vi "Send Launch Nested Panel.vi"(4 "Auto-stop? (T)":bool=TRUE, 6 "timeout in ms (-1)":i32=-1, 7 "Priority":T1=enum."Normal" caption="Message Priority (Normal)", 8 "Error In":errorcluster, 9 "Panel":refnum<class "Panel.lvclass">, 10 "Nested Panel Actor":refnum<class "Panel Actor.lvclass">, 11 "Self Enqueuer in":refnum<class "Message Enqueuer.lvclass">) -> (0 "Error Out":errorcluster, 1 "timed out?":bool, 2 "Nested Actor's Enqueuer":refnum<class "Message Enqueuer.lvclass">)   [LabVIEW 2017, in "MGI-Panel Actor.lvlib" / "Panel Actor.lvclass"]
doc: "Sends a message to the actor to launch a nested panel.\n\n<B>Self Enqueuer In:</B> Enqueuer to send the nested panel message\n<B>Nested Panel Actor:</B> Panel actor to launch as a nested actor.\n<B>Panel:</B> Panel object for displaying the nested Panel Actor.\n<B>timeout in ms (-1):</B> Sets the timeout for launching the nested actor\n<B>Message Priority:</B> Sets the priority for the message.\n<B>Auto-Stop?:</B> Defines if the actor should stop automatically.\n<B>Error In:</B> Describes error conditions that occur before this node runs.\n\n<B>Nested Actor's Enqueuer:</B> Enqueuer for the newly spawned nested actor.\n<B>timed out?</B> Indicates if the action timed out.\n<B>Error Out:</B> Contains error information.\n----\nCopyright: MGI 2018\nAuthor: Derek Trepanier"
uses:
  Panel Actor.lvclass
  <vilib>/ActorFramework/Message Enqueuer/Message Enqueuer.lvclass
  <vilib>/ActorFramework/Message Enqueuer/Message Priority.ctl
  panel-manager/Source/Panel/Panel.lvclass
  Panel Actor Messages/Launch Nested Panel Message Msg/Launch Nested Panel Message Msg.lvclass
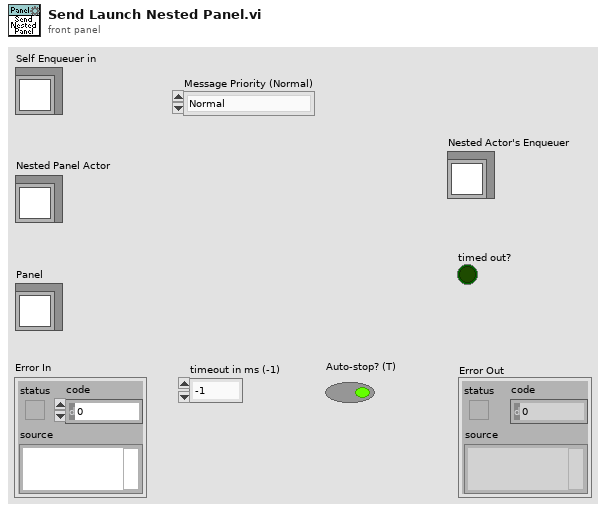
[diagram p1: front panel]
types:
  T1 = typedef "Actor Framework.lvlib/Message Enqueuer.lvclass/Message Priority.ctl" = enum16{"Low", "Normal", "High"}
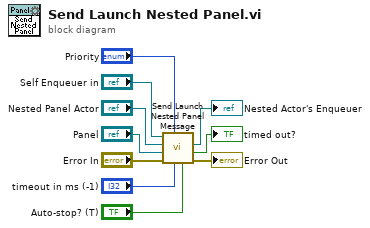
[diagram p0: block diagram]
diagram:
  n1 = call "Send Launch Nested Panel Message.vi"("Auto-stop? (T)"="Auto-stop? (T)", "timeout in ms (-1)"="timeout in ms (-1)", "Priority"="Priority", "error in (no error)"="Error In", "Panel"="Panel", "Nested Panel Actor"="Nested Panel Actor", "Message Enqueuer in"="Self Enqueuer in") -> ("error out"=→"Error Out":errorcluster, "timed out?"=→"timed out?":bool, "Nested Actor's Q"=→"Nested Actor's Enqueuer":refnum<class "Message Enqueuer.lvclass">)  [unwired: 2 in]
